vi "EMAPRE_NOTIF2.vi"(4 "Body":string, 6 "Subject":string, 10 "Password":string, 11 "Email":string) -> ()   [LabVIEW 2015]
uses:
  <vilib>/smtpClient/Set Message Text.vi
  <vilib>/smtpClient/LabVIEWSMTPClient.lvlib
panel:
  in  "To:":string
  in  "TLS":bool=TRUE
  in  "Outgoing Mail Server (SMTP)":string="smtp.gmail.com"
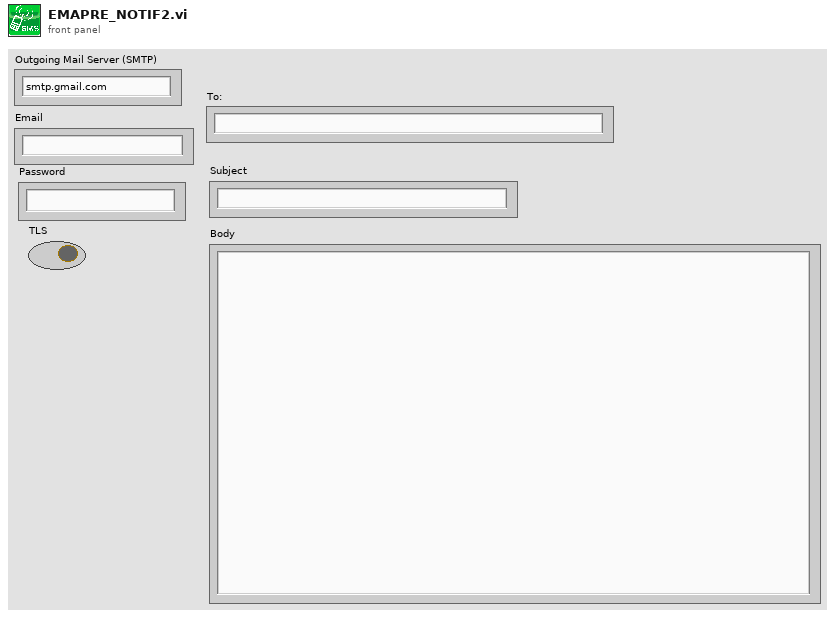
[diagram p1: front panel]
types:
  T1 = typedef "LabVIEWSMTPClient.lvlib/SmtpClientHandle.ctl" = refnum<k1>
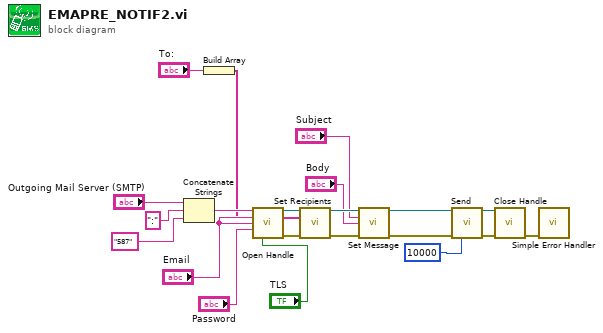
[diagram p0: block diagram]
diagram:
  n1 = Concatenate Strings("Outgoing Mail Server (SMTP)", ":" ("string"), "587" ("Port")) -> (w6:string)
  n2 = Build Array("To:") -> (w1:string[])
  n3 = call <vilib>:"Open Handle.vi"("server address"=w6, "from"="Email", "username"="Email", "password"="Password", "use TLS (false)"="TLS") -> ("handle out"=w21:T1, "error out"=w18:errorcluster)  [unwired: 9 in]
  n4 = call <vilib>:"Set Recipients.vi"("handle in"=w21, "to"=w1, "error in (no error)"=w18) -> ("handle out"=w17:T1, "error out"=w16:errorcluster)  [unwired: 11 in]
  n5 = call-poly <vilib>:"Set Message.vi"("handle in"=w17, "subject"="Subject", "plain text message"="Body", "error in (no error)"=w16) -> ("handle out"=w13:T1, "error out"=w12:errorcluster)  [unwired: 10 in]
  n6 = call <vilib>:"Send.vi"("handle in"=w13, "error in (no error)"=w12, "timeout in ms (10000)"=10000) -> ("handle out"=w11:T1, "error out"=w10:errorcluster)  [unwired: 10 in, 1 out]
  n7 = call <vilib>:"Close Handle.vi"("handle in"=w11, "error in (no error)"=w10) -> ("error out"=w3:errorcluster)  [unwired: 12 in, 1 out]
  n8 = call <vilib>:"Simple Error Handler.vi"("error in (no error)"=w3) -> ()  [unwired: 4 in, 5 out]
